vi "Global - Monitoring Variables.vi"() -> ()   [LabVIEW 2014]
uses:
  controls/FPGA VI Reference.ctl
panel:
  out "ADCs Current Value":dbl[](array[numeric])
  in  "Current FPGA VI Reference":T1
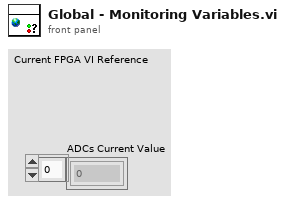
[diagram p1: front panel]
types:
  T1 = typedef "FPGA VI Reference.ctl" = refnum<k20>
diagram:
